vi "俄罗斯方块.vi"() -> ()   [LabVIEW 2018]
panel:
  in  "停止":bool
  out "分数":string
  out "等级":string
  in  "数组 3":bool[][](array[boolean])
  out "?":bool[][](array[boolean])
  # "下一个"
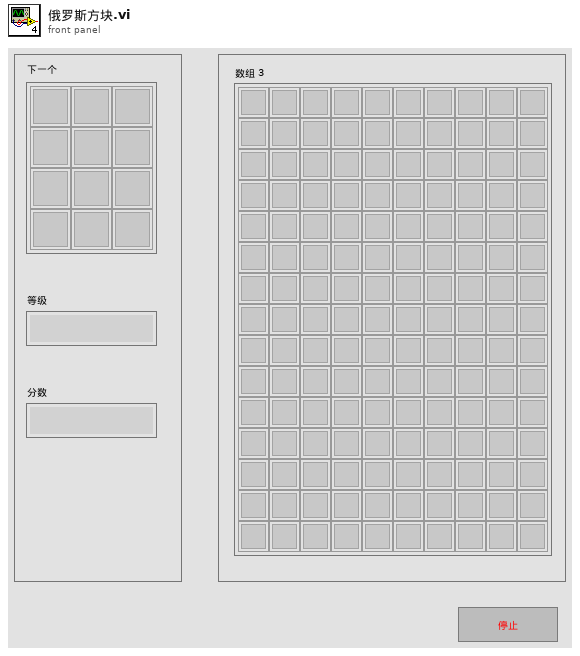
[diagram p1: front panel]
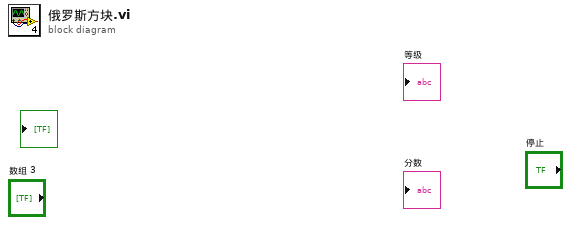
[diagram p0: block diagram]
diagram:
